vi "Lookup Description.vi"(8 "error in (no error)":errorcluster, 10 "Tree Tag":string, 11 "Message Maker in":refnum<class "Message Maker.lvclass">) -> (0 "error out":errorcluster, 2 "Description":string, 3 "Message Maker out":refnum<class "Message Maker.lvclass">)   [LabVIEW 2023, in "Message Maker.lvclass"]
doc: "Given a tag, looks up the description field\n\nAuthor: Derek Trepanier\nCopyright: MGI 2015"
uses:
  Message Maker.lvclass
  Message Maker.lvclass/Message Maker.ctl
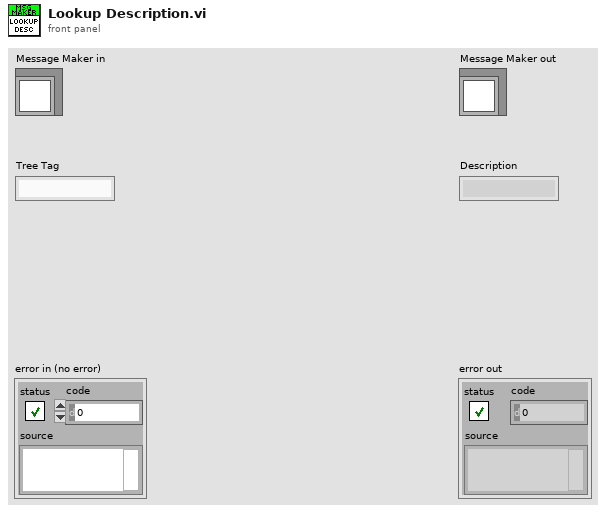
[diagram p1: front panel]
types:
  T1 = typedef "Message Maker.lvclass/Details Map.ctl" = map{string, string}
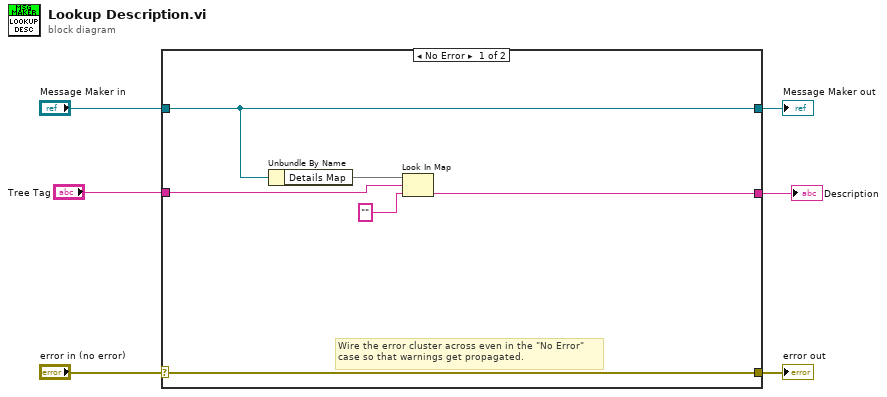
[diagram p0: block diagram]
diagram:
  n1 = case shown="No Error" "error in (no error)" {
    selector: "error in (no error)" -> [w12 w14]
    tunnel: [w12 w14] -> w5
    tunnel: [w11 w13] -> w3
    tunnel: "Message Maker in" -> [w11 w13]
    tunnel: "Tree Tag" -> [w9 _]
    tunnel: [w7 _] -> w1
    frame No Error {
      # "Wire the error cluster across even in the \"No Error\"\ncase so that warnings get propagated."
      n2 = Unbundle By Name(w11) -> ("Details Map"=w10:T1)
      n3 = Look In Map(map=w10, key=w9, default value="" ("Tree Tag")) -> (value=w7:string)  [unwired: 1 out]
    }
    frame Error {
    }
  }
  "error out" <- w5
  "Message Maker out" <- w3
  "Description" <- w1
